vi "Get cif_channelcore_ChannelFilter.vi"(8 "error in (no error)":errorcluster, 11 "gRPCid":T1) -> (0 "error out":errorcluster, 2 "package_templatemessage":T2, 3 "gRPCid out":T1)   [LabVIEW 2021, in "CIFCoreChannel_server.lvlib"]
uses:
  CIFCoreChannel_server.lvlib
  cif_channelcore_ChannelFilter.ctl
  cif_channelcore_ChannelDirection.ctl
  <vilib>/gRPC/LabVIEW gRPC Library/Shared/grpcId.ctl
  cif_channelcore_ChannelFilter_Flat.ctl
  2ed25e12-861d-4677-8ead-ace2906b2041.vi
  <vilib>/gRPC/LabVIEW gRPC Library/Shared/TranslateGrpcError.vi
  <vilib>/gRPC/LabVIEW gRPC Library/Server API/Server/Get Server DLL Path.vi
  <vilib>/Utility/error.llb/Error Cluster From Error Code.vi
  <vilib>/gRPC/LabVIEW gRPC Library/grpc-lvsupport-release.lvlib
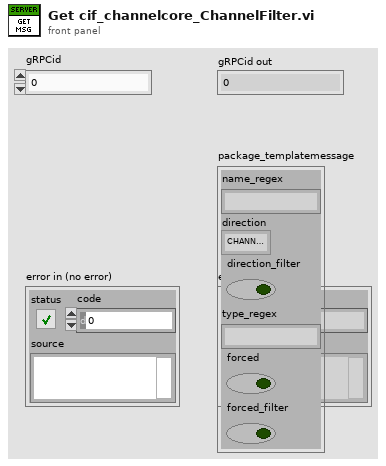
[diagram p1: front panel]
types:
  T1 = typedef "grpc-lvsupport-release.lvlib/grpcId.ctl" = u64
  T2 = typedef "CIFCoreChannel_server.lvlib/cif_channelcore_ChannelFilter.ctl" = cluster{"name_regex":string, "direction":T3, "direction_filter":bool, "type_regex":string, "forced":bool, "forced_filter":bool}
  T3 = typedef "CIFCoreChannel_server.lvlib/cif_channelcore_ChannelDirection.ctl" = enum32{"CHANNELDIRECTION_UNKNOWN", "CHANNELDIRECTION_PUBLISHER", "CHANNELDIRECTION_SUBSCRIBER"}
  T4 = typedef "CIFCoreChannel_server.lvlib/cif_channelcore_ChannelFilter_Flat.ctl" = cluster{"name_regex":string, "direction":T3, "direction_filter":bool, "type_regex":string, "forced":bool, "forced_filter":bool}
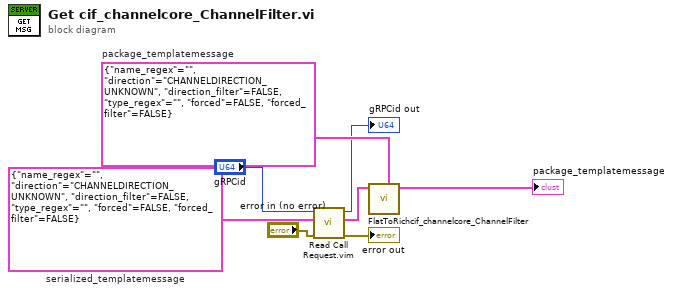
[diagram p0: block diagram]
diagram:
  w6 = T4 {"name_regex"="", "direction"=enum."CHANNELDIRECTION_UNKNOWN", "direction_filter"=FALSE, "type_regex"="", "forced"=FALSE, "forced_filter"=FALSE}  # serialized_templatemessage
  w5 = T2 {"name_regex"="", "direction"=enum."CHANNELDIRECTION_UNKNOWN", "direction_filter"=FALSE, "type_regex"="", "forced"=FALSE, "forced_filter"=FALSE}  # package_templatemessage
  n1 = call "Read Call Request.vim"("error in"="error in (no error)", "Request Type"=w6, "gRPCid in"="gRPCid") -> ("error out"=→"error out":errorcluster, "Request Data"=w4:T4, "gRPCid out"=→"gRPCid out":T1)  [unwired: 6 in]
  n2 = call "FlatToRichcif_channelcore_ChannelFilter.vi"("OutputClusterType"=w5, "InputCluster"=w4) -> ("OutputCluster"=→"package_templatemessage":T2)  [unwired: 9 in]
